vi "LeakageDetector.vi"(2 "error in (no error)":errorcluster) -> (0 "error out":errorcluster)   [LabVIEW 2013]
uses:
  My Computer/Controls/Sensors State.ctl
  <vilib>/myRIO/Instrument Drivers/Onboard IO/AI/vis/Smart Open.vi
  <vilib>/myRIO/Instrument Drivers/Onboard IO/AI/vis/Read.vi
  <vilib>/myRIO/Instrument Drivers/Onboard IO/AI/vis/Open.vi
  <vilib>/myRIO/Common/Instrument Driver Framework/myRIO v1.0/AI/vis/myRIO v1.1 Open AI.vi
  <vilib>/myRIO/Common/Instrument Driver Framework/Utilities/vis/Validate Channels.vi
  <vilib>/myRIO/Common/Instrument Driver Framework/myRIO v1.0/AI/vis/myRIO v1.0 Reserve AI.vi
  <vilib>/myRIO/Common/Instrument Driver Framework/myRIO v1.0/AI/vis/myRIO v1.0 Build MUX Configuration AI.vi
  <vilib>/myRIO/Common/Instrument Driver Framework/myRIO v1.0/Resource Manager/vis/myRIO v1.0 Reserve Channel List.vi
  <vilib>/myRIO/Common/Instrument Driver Framework/myRIO v1.0/Resource Manager/vis/myRIO v1.0 Reserve Channel.vi
  <vilib>/myRIO/Common/Instrument Driver Framework/myRIO v1.0/Resource Manager/vis/myRIO v1.0 Unreserve Channel.vi
  <vilib>/myRIO/Common/Instrument Driver Framework/myRIO v1.0/Resource Manager/vis/myRIO v1.0 Build Mutex Name.vi
  <vilib>/myRIO/Common/Instrument Driver Framework/myRIO v1.0/myRIO v1.1 Open.vi
  <vilib>/myRIO/Common/Instrument Driver Framework/myRIO v1.0/AI/vis/myRIO v1.0 Get Scaling Constants AI.vi
  <vilib>/Utility/VariantDataType/GetNumericInfo.vi
  <vilib>/Utility/error.llb/Error Cluster From Error Code.vi
  <vilib>/myRIO/Common/Instrument Driver Framework/Utilities/vis/IO Manager.vi
  <vilib>/myRIO/Common/Instrument Driver Framework/Utilities/vis/Configuration Manager.vi
  <vilib>/myRIO/Common/Instrument Driver Framework/myRIO v1.0/myRIO v1.0 Close.vi
  <vilib>/myRIO/Common/Instrument Driver Framework/myRIO v1.0/AI/vis/myRIO v1.0 Read AI.vi
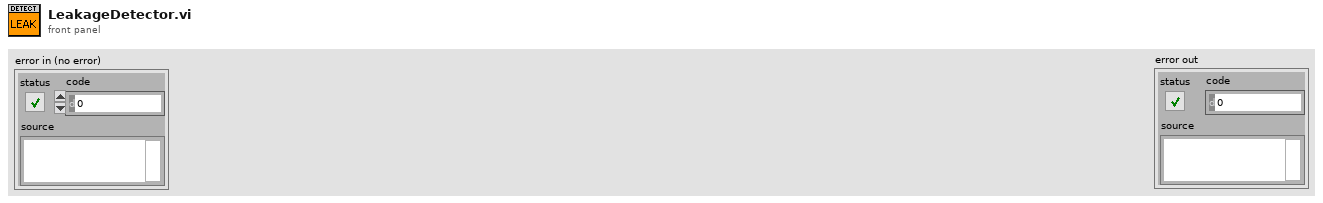
[diagram p1: front panel]
types:
  T1 = typedef "Sensors State.ctl" = cluster{"Leakage-Sensor_enabled":bool, "IMU_enabled":bool, "Swimbladder Fill-State-Sensor_enabled":bool, "Flow-Sensor_enabled":bool, "Depth-Sensor_enabled":bool, "Current-Sensor_enabled":bool, "Calibrate Depth":bool, "SB_Piston_Stuck_Detect_enabled":bool, "Check_too_Deep_enabled":bool}
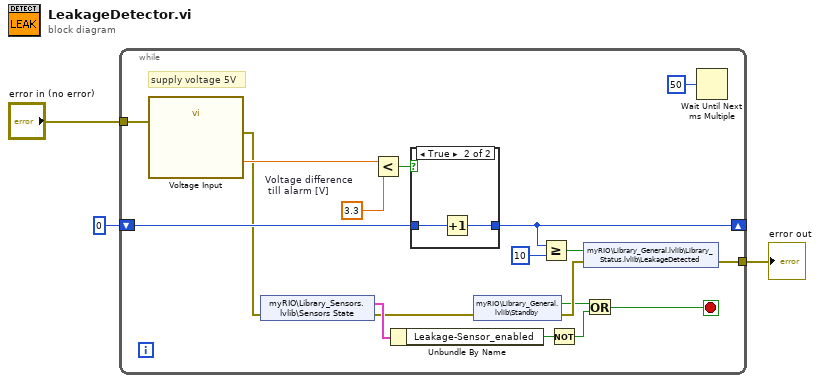
[diagram p0: block diagram]
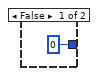
[diagram p2: hidden frame]
diagram:
  n1 = while {
    tunnel: "error in (no error)" -> [w11]
    tunnel: [w18] -> w1
    shift-right: [w7] -> _
    shift-left: 0 -> [w8]
    stop <- w16 stop-if-true
    w21 = 3.3  # Voltage difference  till alarm [V]
    # "supply voltage 5V"
    n2 = call "Voltage Input"("error in (no error)"=w11) -> ("VOUT Leakage (A/AI0 (Pin 3))"=w17:dbl, "error out"=w4:errorcluster)  [unwired: 25 in]
    n3 = shared-variable "myRIO\\Library_Sensors.lvlib\\Sensors State"(error in=w4) -> (w13:T1, error out=w10:errorcluster)
    n4 = Less?(x=w17, y=w21) -> (x < y?=w9:bool)
    n5 = Unbundle By Name(w13) -> ("Leakage-Sensor_enabled"=w12:bool)
    n6 = case shown="True" w9 {
      tunnel: w8 -> [_ w24]
      tunnel: [0 w23] -> w7
      frame False {
      }
      frame True {
        n7 = Increment(x=w24) -> (x+1=w23:i32)
      }
    }
    n8 = shared-variable "myRIO\\Library_General.lvlib\\Standby"(error in=w10) -> (w15:bool, error out=w19:errorcluster)
    n9 = Greater Or Equal?(x=w7, y=10) -> (x >= y?=w5:bool)
    n10 = Not(x=w12) -> (.not. x?=w14:bool)
    n11 = shared-variable "myRIO\\Library_General.lvlib\\Library_Status.lvlib\\LeakageDetected"(w5, error in=w19) -> (error out=w18:errorcluster)
    n12 = Or(x=w15, y=w14) -> (x .or. y?=w16:bool)
    n13 = Wait Until Next ms Multiple(millisecond multiple=u32 50) -> ()  [unwired: 1 out]
  }
  "error out" <- w1
